vi "ECG_WriteFile.vi"(7 "ECG waveform data":i64[](array[numeric]) caption="ECG 波形数据", 8 "error in (no error)":errorcluster caption="错误输入（无错误）", 10 "patient ID":string caption="病人 ID", 11 "ECG waveform file path":string caption="ECG 波形文件路径") -> (0 "error out":errorcluster caption="错误输出", 2 "ECG new file name":string caption="ECG 新建波形文件名称", 3 "ECG waveform new file path":path caption="ECG 新建波形文件路径")   [LabVIEW 2022 SP3]
uses:
  <vilib>/Utility/file.llb/Write Delimited Spreadsheet (I64).vi
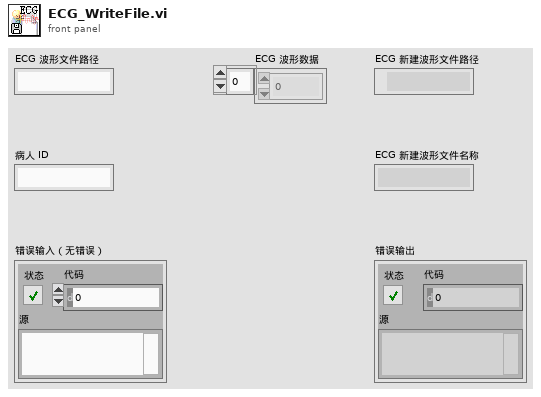
[diagram p1: front panel]
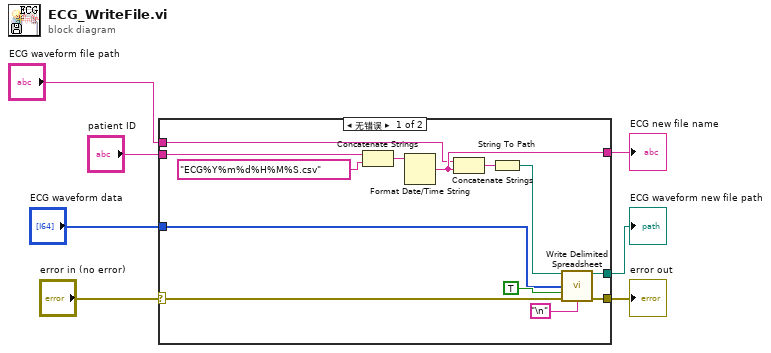
[diagram p0: block diagram]
diagram:
  n1 = case shown="无错误" "error in (no error)" {
    selector: "error in (no error)" -> [w8 w21]
    tunnel: [w20 _] -> w7
    tunnel: "patient ID" -> [w19 _]
    tunnel: [w18 _] -> w5
    tunnel: [w15 w21] -> w4
    tunnel: "ECG waveform file path" -> [w12 _]
    tunnel: "ECG waveform data" -> [w9 _]
    frame No Error {
      n2 = Concatenate Strings(w19, "ECG%Y%m%d%H%M%S.csv" ("时间格式字符串(%c)")) -> (w17:string)
      n3 = Format Date/Time String(time format string (%c)=w17) -> (date/time string=w18:string)  [unwired: 2 in]
      n4 = Concatenate Strings(w12, w18) -> (w13:string)
      n5 = String To Path(string=w13) -> (path=w14:path)
      n6 = call-poly <vilib>:"Write Delimited Spreadsheet.vi"("file path (dialog if empty)"=w14, "1D data"=w9, "append to file? (new file:F)"=TRUE, "error in (no error)"=w8, "delimiter (\\t)"="\n" ("delimiter (\\t)")) -> ("new file path (Not A Path if cancelled)"=w20:path, "error out"=w15:errorcluster)  [unwired: 9 in]
    }
    frame Error {
    }
  }
  "ECG waveform new file path" <- w7
  "ECG new file name" <- w5
  "error out" <- w4
